vi "Run Sequences.vi"(8 "error in (no error)":errorcluster, 10 "Error Notifier in":refnum<notifier>, 11 "Sequence Queue in":refnum<queue>) -> (0 "error out":errorcluster)   [LabVIEW 2015, in "Mediator.lvlib" / "Mediator.lvclass"]
doc: "This VI executes enqueued sequences. It is run as a background process by the Mediator."
uses:
  Mediator.lvclass
  Sequence/Sequence.lvclass
  Controls/Sequence Error.ctl
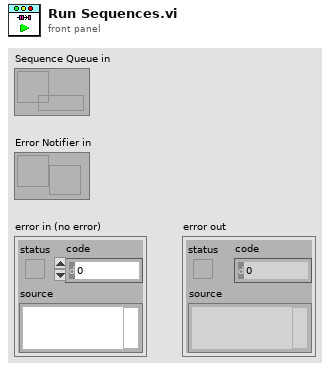
[diagram p1: front panel]
types:
  T1 = typedef "Mediator.lvlib/Sequence.lvclass/Sequence Error.ctl" = cluster{"Name":string, "Error Out":errorcluster}
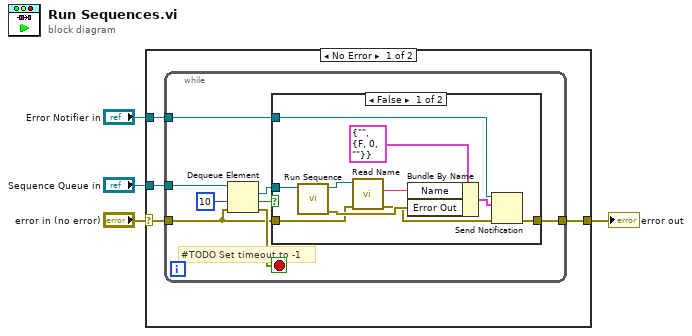
[diagram p0: block diagram]
diagram:
  n1 = case shown="No Error" "error in (no error)" {
    selector: "error in (no error)" -> [w8 w28]
    tunnel: [w7 w28] -> w3
    tunnel: "Sequence Queue in" -> [w6 _]
    tunnel: "Error Notifier in" -> [w5 _]
    frame No Error {
      n2 = while {
        tunnel: w8 -> [w9]
        tunnel: [w13] -> w7
        tunnel: w6 -> [w11]
        tunnel: w5 -> [w10]
        stop <- w12 stop-if-true
        # "#TODO Set timeout to -1"
        n3 = Dequeue Element(queue=w11, timeout in ms (-1)=10, error in (no error)=w9) -> (element=w14:refnum<class "Sequence.lvclass">, timed out?=w15:bool, error out=w12:errorcluster)  [unwired: 1 out]
        n4 = case shown="False" w15 {
          tunnel: w14 -> [w23 _]
          tunnel: w9 -> [w18 w27]
          tunnel: [w26 w27] -> w13
          tunnel: w10 -> [w24 _]
          frame False {
            n5 = call-dynamic "Run Sequence.vi"("Sequence in"=w23) -> ("error out"=w21:errorcluster, "Sequence out"=w20:refnum<class "Sequence.lvclass">)  [unwired: 9 in]
            n6 = call-dynamic "Read Name.vi"("error in (no error)"=w18, "Sequence in"=w20) -> ("error out"=w19:errorcluster, "Name"=w22:string)  [unwired: 7 in, 1 out]
            n7 = Bundle By Name(cluster=T1 {"Name"="", "Error Out"={"status"=FALSE, "code"=0, "source"=""}} ("notification"), "Name"=w22, "Error Out"=w21) -> (w17:T1)
            n8 = Send Notification(notification=w17, notifier=w24, error in (no error)=w19) -> (error out=w26:errorcluster)  [unwired: 1 out]
          }
          frame True {
          }
        }
      }
    }
    frame Error {
    }
  }
  "error out" <- w3
